vi "Send Binary Decision Msg Reply.vi"(8 "Error In":errorcluster, 11 "BinaryDecisionMsg in":refnum<class "BinaryDecisionMsg.lvclass">) -> (0 "error out":errorcluster)   [LabVIEW 2017, in "AbstractMessages.lvlib" / "BinaryDecisionMsg.lvclass"]
uses:
  BinaryDecisionMsg.lvclass
  C:/Git/mva-framework/Framework/AbstractMessages/PreAddressedMsg/PreAddressedMsg.lvclass
  PreAddressedMsg/PreAddressedMsg.lvclass/PreAddressedMsg.ctl
  BinaryDecisionMsg.lvclass/BinaryDecisionMsg.ctl
  <vilib>/ActorFramework/Message Enqueuer/Message Enqueuer.lvclass/Message Enqueuer.ctl
  <vilib>/ActorFramework/Message Priority Queue/Priority Enqueue.vi
  PreAddressedMsg/PreAddressedMsg.lvclass
  <vilib>/ActorFramework/Message Enqueuer/Message Enqueuer.lvclass
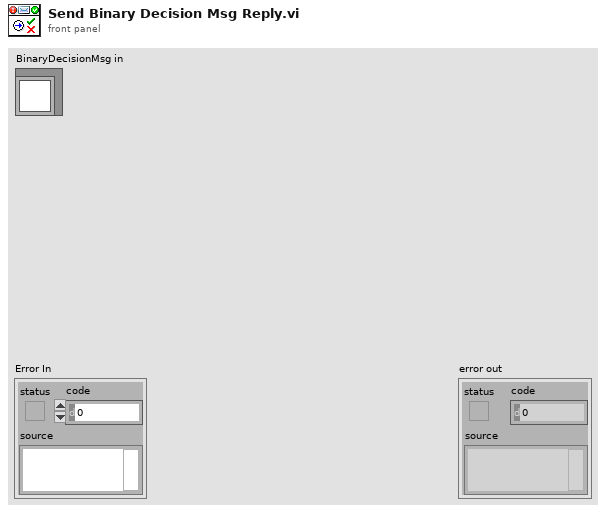
[diagram p1: front panel]
types:
  T1 = typedef "Actor Framework.lvlib/Message Enqueuer.lvclass/Message Priority.ctl" = enum16{"Low", "Normal", "High"}
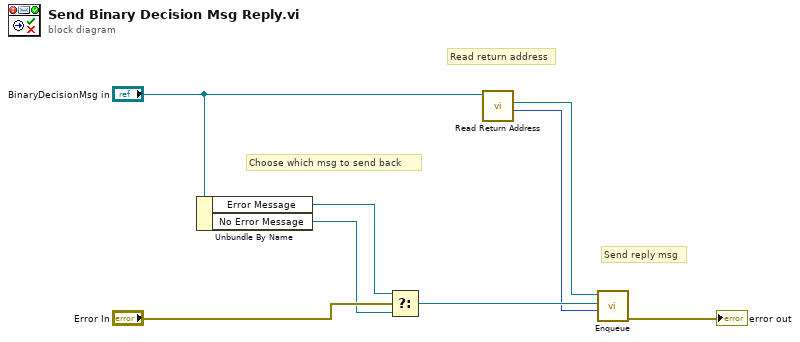
[diagram p0: block diagram]
diagram:
  # "Send reply msg"
  # "Read return address"
  # "Choose which msg to send back"
  n1 = Unbundle By Name("BinaryDecisionMsg in") -> ("Error Message"=w4:refnum<class "Message.lvclass">, "No Error Message"=w3:refnum<class "Message.lvclass">)
  n2 = Select(t=w4, s="Error In", f=w3) -> (s? t:f=w2:refnum<class "Message.lvclass">)
  n3 = call "Read Return Address.vi"("PreAddressedMsg in"="BinaryDecisionMsg in") -> ("Return Priority (Normal)"=w1:T1, "Return Address"=w7:refnum<class "Message Enqueuer.lvclass">)  [unwired: 9 in]
  n4 = call <vilib>:"Enqueue.vi"("Message Priority (Normal)"=w1, "Message"=w2, "Message Enqueuer in"=w7) -> ("error out"=→"error out":errorcluster)  [unwired: 7 in, 1 out]
